vi "Actor Core.vi"(8 "error in":errorcluster, 11 "SDO Manager Worker in":refnum<class "Response Matcher.lvclass">) -> (0 "error out":errorcluster, 3 "Actor out":refnum<class "Actor.lvclass">)   [LabVIEW 2020, in "CANopen.lvlib" / "Response Matcher.lvclass"]
doc: "<p>(<strong>Filename</strong>: <span class=\"dnl\">Actor Framework.lvlib:Actor.lvclass:Actor Core.vi</span>)</p>\n<p>Receives messages to the actor, reacts to them, and initiates any error handling that may shut the actor down.</p>\n<p>Descendant classes may override this VI to append parallel tasks for the actor to complete while it handles messages. Overrides use the <a href=\"nihelplauncher://docs/csh?context=lvcore_glang_udclass\">Call Parent Class Method</a> node.</p>"
uses:
  Response Matcher.lvclass
  <vilib>/ActorFramework/Actor/Actor.lvclass
  Response Matcher.lvclass/Response Matcher.ctl
  HAL/Source/Interfaces/ICAN CC Frame/ICAN CC Frame.lvclass
  SDO Transfer/SDO Transfer.lvclass
  Logging/Log Level.vi
  Logging/CANopen Logging.lvlib
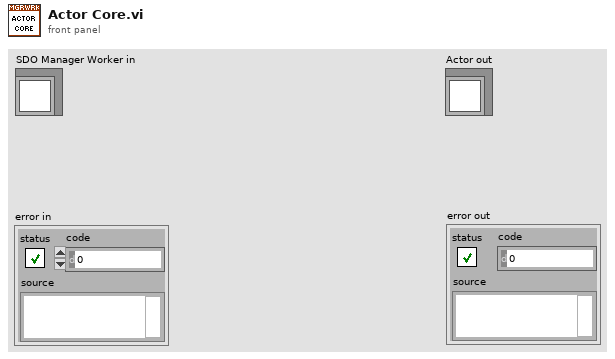
[diagram p1: front panel]
types:
  T1 = enum16{"Error", "Warn", "Info", "Debug", "Trace"}
  T2 = map{string, refnum<class "SDO Transfer.lvclass">}
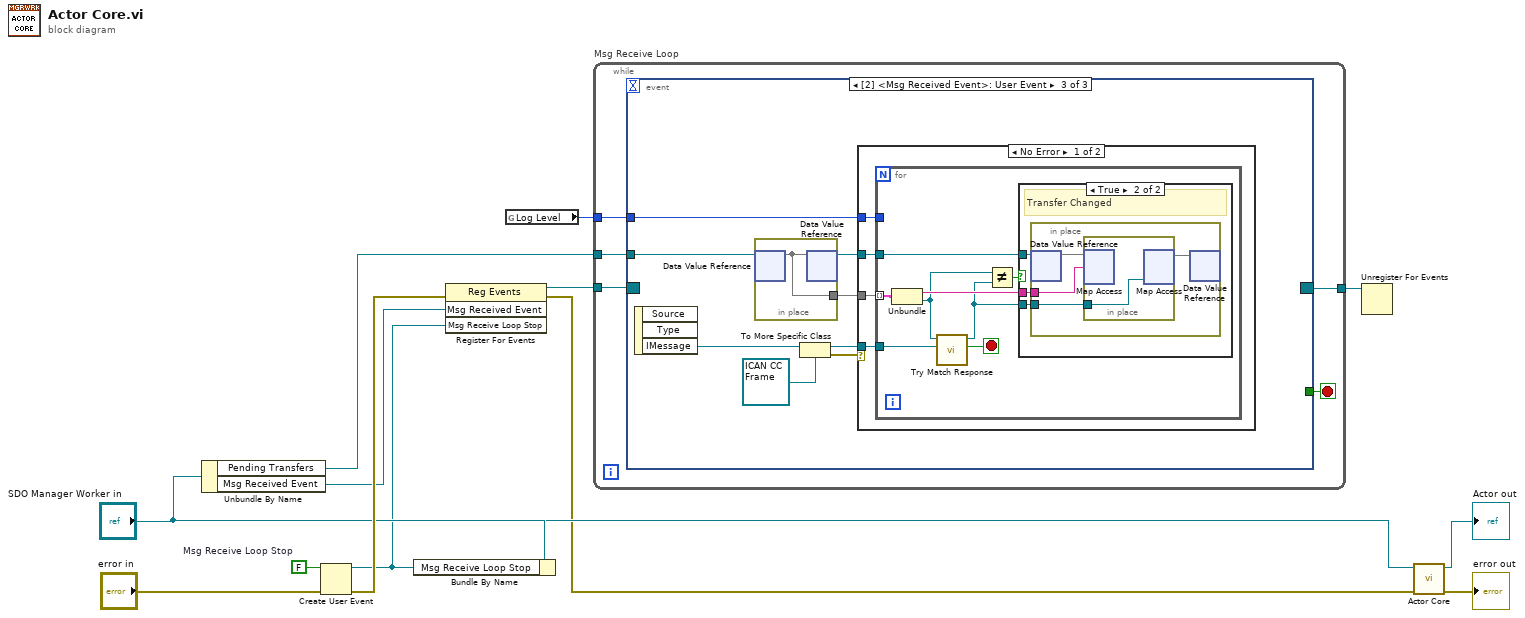
[diagram p0: block diagram]
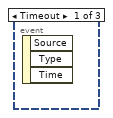
[diagram p2: hidden frame]
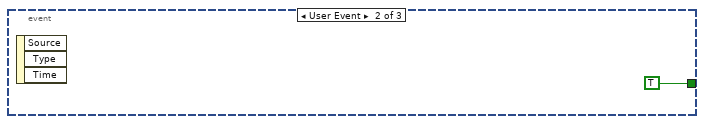
[diagram p3: hidden frame]
diagram:
  w10 = FALSE  # Msg Receive Loop Stop
  n1 = Unbundle By Name("SDO Manager Worker in") -> ("Pending Transfers"=w4:refnum<data-value>, "Msg Received Event"=w8:refnum<user-event>)
  n2 = Create User Event(user event datatype=w10, error in="error in") -> (user event=w7:refnum<user-event>, error out=w14:errorcluster)
  n3 = Bundle By Name(cluster="SDO Manager Worker in", "Msg Receive Loop Stop"=w7) -> (w5:refnum<class "Response Matcher.lvclass">)
  n4 = register-events(error in=w14, w8, w7) -> (reference out=w2:refnum<event-registration>, error out=w3:errorcluster)  [unwired: 1 in]
  n5 = global read "Log Level.vi" "Log Level"() -> (w1:T1)
  n6 = while "Msg Receive Loop" {
    tunnel: w2 -> [w18]
    tunnel: [w17] -> w6
    tunnel: w4 -> [w16]
    tunnel: w1 -> [w15]
    stop <- w19 stop-if-true
    n7 = event shown="[2] <Msg Received Event>: User Event" {
      selector: w18 -> [_ _ _]
      dyn-events: [_ _ _] -> w17
      timeout: _ -> [_ _ _]
      tunnel: [_ TRUE _] -> w19
      tunnel: w16 -> [_ _ w21]
      tunnel: w15 -> [_ _ w27]
      event Timeout {
        n8 = event-data() -> ()  [unwired: 1 in, 3 out]
      }
      event User Event {
        n9 = event-data() -> ()  [unwired: 1 in, 3 out]
      }
      event User Event {
        n10 = event-data() -> ("IMessage"=w28:refnum<class "IMessage.lvclass">)  [unwired: 1 in, 2 out]
        n11 = in-place {
          in-place-border: [w49] -> w26
          n12 = in-place-dvr #1(w21) -> (w49:T2)  [unwired: 1 out]
          n13 = in-place-dvr #1(w49) -> (w22:refnum<data-value>)  [unwired: 1 out]
        }
        n14 = To More Specific Class(target class=refnum<class "ICAN CC Frame.lvclass"> refnum ("ICAN CC Frame"), reference=w28) -> (specific class reference=w25:refnum<class "ICAN CC Frame.lvclass">, error out=w23:errorcluster)  [unwired: 1 in]
        n15 = case shown="No Error" w23 {
          tunnel: w26 -> [w32 _]
          tunnel: w25 -> [w31 _]
          tunnel: w27 -> [w30 _]
          tunnel: w22 -> [w29 _]
          frame No Error {
            n16 = for {
              tunnel: w32 -> [w40] mode=indexing
              tunnel: w31 -> [w39]
              tunnel: w30 -> [_]
              tunnel: w29 -> [w37]
              stop <- w38 stop-if-true
              n17 = Unbundle(w40) -> ("NI GUID"=w36:string, "SDO Transfer"=w33:refnum<class "SDO Transfer.lvclass">)
              n18 = call-dynamic "Try Match Response.vi"("ICAN CC Frame"=w39, "SDO Transfer in"=w33) -> ("Success"=w38:bool, "SDO Transfer out"=w34:refnum<class "SDO Transfer.lvclass">)  [unwired: 7 in, 1 out]
              n19 = Not Equal?(x=w33, y=w34) -> (x != y?=w35:bool)
              n20 = case shown="True" w35 {
                tunnel: w37 -> [_ w43]
                tunnel: w36 -> [_ w42]
                tunnel: w34 -> [_ w41]
                frame False {
                  # "Transfer Unchanged"
                }
                frame True {
                  # "Transfer Changed"
                  n21 = in-place {
                    in-place-border: w42 -> [w45]
                    in-place-border: w41 -> [w44]
                    n22 = in-place-dvr #2(w43) -> (w47:T2)  [unwired: 1 out]
                    n23 = in-place {
                      in-place-border: w44 -> [w48]
                      n24 = in-place-map #3(w47, w45) -> ()  [unwired: 1 in, 2 out]
                      n25 = in-place-map #3(w48) -> (w46:T2)  [unwired: 1 in, 2 out]
                    }
                    n26 = in-place-dvr #2(w46) -> ()  [unwired: 2 out]
                  }
                }
              }
            }
          }
          frame Error {
          }
        }
      }
    }
  }
  n27 = Unregister For Events(event registration refnum=w6) -> ()  [unwired: 1 in, 1 out]
  n28 = call-parent "Actor Core.vi"("error in"=w3, "Actor in"=w5) -> ("error out"=→"error out":errorcluster, "Actor out"=→"Actor out":refnum<class "Actor.lvclass">)  [unwired: 8 in]
